vi "pelletron voltage update.vi"(0 "Enable":bool=TRUE, 5 "error in (no error)":errorcluster) -> (14 "Cancel":bool caption="OK", 17 "Pelletron Voltage":dbl format="%#g", 18 "Continue":bool caption="OK", 19 "error out":errorcluster)   [LabVIEW 2012]
doc: "Displays a standard dialog box that prompts users to enter information, such as a user name and password.\n--------------------\n\nThis Express VI is configured as follows:\n\nMessage to Display to the User:Please enter the following pelletron data:\nThe inputs are: \nNumber: Pelletron Voltage"
panel:
  in  "Pelletron Voltage (MV):":dbl caption="Pelletron Voltage" min=0.0 max=3.299999952316284 format="%#g"
  out "String":string="Please enter the following pelletron data:"
  in  "Cancel":bool
  in  "OK2":bool
  in  "OK1":bool
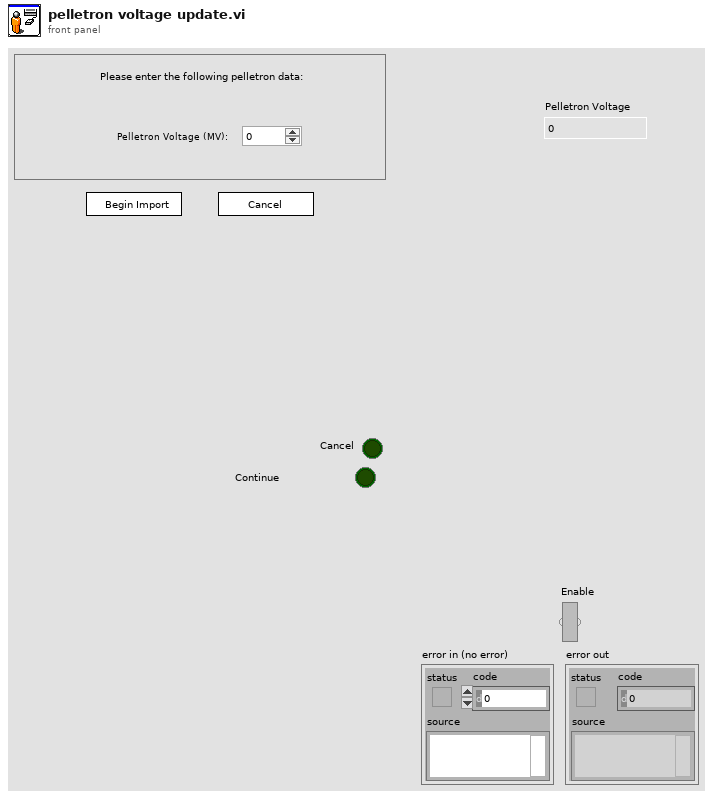
[diagram p1: front panel]
types:
  T1 = cluster{"Input Name":string, "Input Data Type":i32}[]
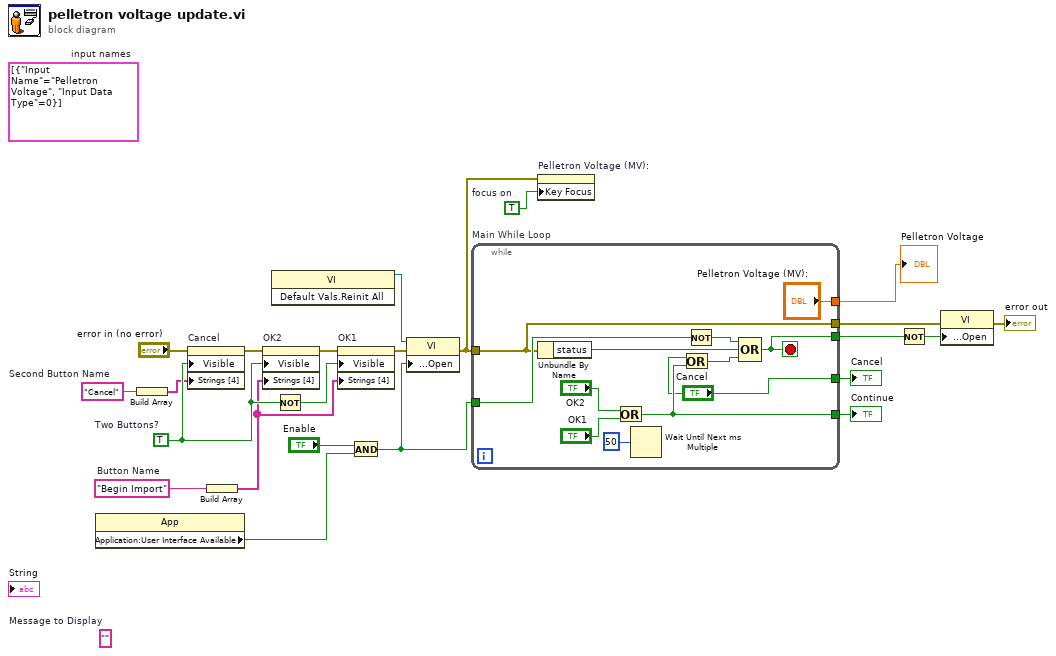
[diagram p0: block diagram]
diagram:
  w2 = TRUE  # focus on
  (unwired) T1 [{"Input Name"="Pelletron Voltage", "Input Data Type"=0}]  # input names
  w15 = "Cancel"  # Second Button Name
  w13 = "Begin Import"  # Button Name
  (unwired) ""  # Message to Display
  w23 = TRUE  # Two Buttons?
  n1 = property class="App"() -> ("Application:User Interface Available"=w5:bool)  [unwired: 2 in, 2 out]
  n2 = Build Array(w15) -> (w16:string[])
  n3 = property on="Cancel" class="Bool"(error in="error in (no error)", "Visible"=w23, "Strings [4]"=w16) -> (error out=w20:errorcluster)  [unwired: 1 in, 1 out]
  n4 = Build Array(w13) -> (w14:string[])
  n5 = property on="OK2" class="Bool"(error in=w20, "Visible"=w23, "Strings [4]"=w14) -> (error out=w19:errorcluster)  [unwired: 1 in, 1 out]
  n6 = invoke class="VI" method="Default Vals.Reinit All"() -> (reference out=w4:refnum<vi>)  [unwired: 3 in, 2 out]
  n7 = Not(x=w23) -> (.not. x?=w21:bool)
  n8 = property on="OK1" class="Bool"(error in=w19, "Visible"=w21, "Strings [4]"=w14) -> (error out=w12:errorcluster)  [unwired: 1 in, 1 out]
  n9 = And(x="Enable", y=w5) -> (x .and. y?=w6:bool)
  n10 = property class="VI"(reference=w4, error in=w12, "Front Panel Window:Open"=w6) -> (error out=w11:errorcluster)  [unwired: 1 out]
  n11 = while "Main While Loop" {
    tunnel: [w33] -> w22
    tunnel: w6 -> [w31]
    tunnel: [w29] -> w17
    tunnel: w11 -> [w28]
    tunnel: [w28] -> w9
    tunnel: ["Pelletron Voltage (MV):"] -> w3
    tunnel: ["Cancel"] -> w1
    stop <- w29 stop-if-true
    n12 = Unbundle By Name(w28) -> ("status"=w26:bool)
    n13 = Or(x="OK2", y="OK1") -> (x .or. y?=w33:bool)
    n14 = Wait Until Next ms Multiple(millisecond multiple=u32 50) -> ()  [unwired: 1 out]
    n15 = Or(x="Cancel", y=w33) -> (x .or. y?=w27:bool)
    n16 = Not(x=w31) -> (.not. x?=w30:bool)
    n17 = Compound Arithmetic op=OR(w30, w26, w27) -> (w29:bool)
  }
  "Continue" <- w22
  "Pelletron Voltage" <- w3
  "Cancel" <- w1
  n18 = property on="Pelletron Voltage (MV):" class="DigNum (strict)"(error in=w11, "Key Focus"=w2) -> ()  [unwired: 1 in, 2 out]
  n19 = Not(x=w17) -> (.not. x?=w18:bool)
  n20 = property class="VI"(error in=w9, "Front Panel Window:Open"=w18) -> (error out=→"error out":errorcluster)  [unwired: 1 in, 1 out]
